vi "PromptWrite.vi"(8 "error in":errorcluster, 9 "time":timestamp, 10 "string":string, 11 "TerminalIn":T1) -> (0 "error out":errorcluster, 3 "TerminalOut":T1)   [LabVIEW 2021, in "LibDan.lvlib"]
uses:
  LibDan.lvlib
  TerminalDef.ctl
  <vilib>/Utility/config.llb/Config Data RefNum.ctl
  <vilib>/Utility/config.llb/NI_LVConfig.lvlib
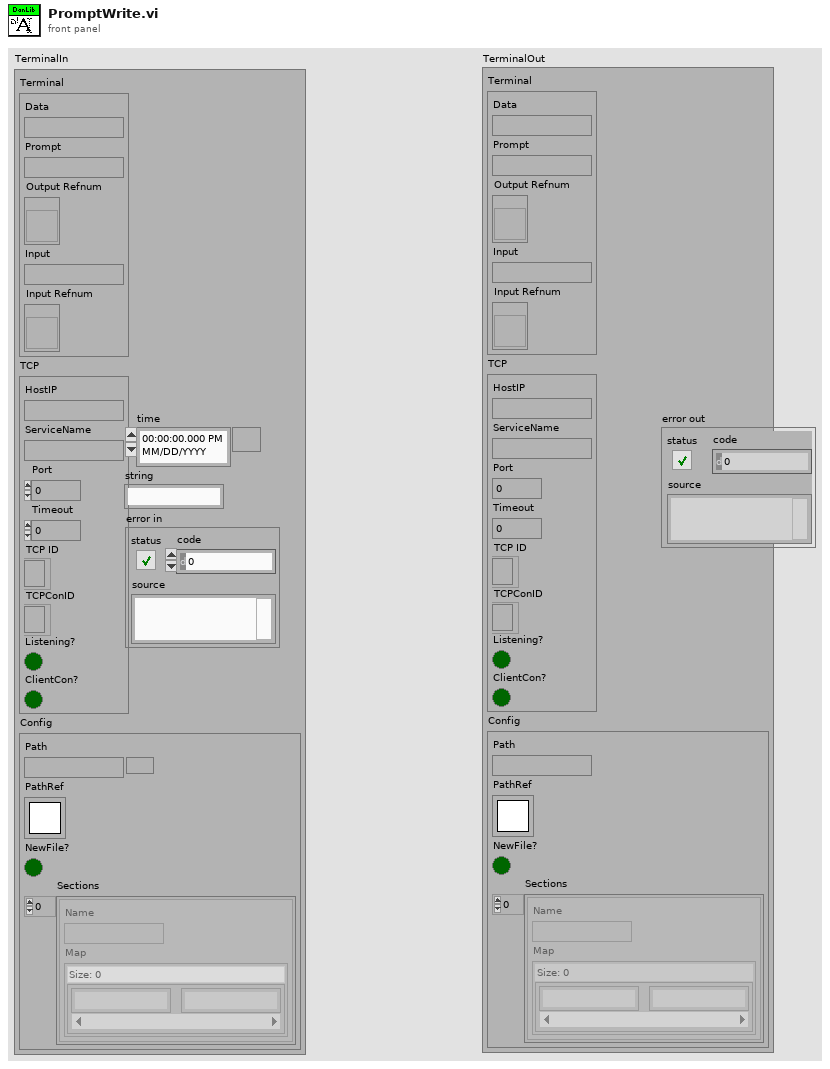
[diagram p1: front panel]
types:
  T1 = typedef "LibDan.lvlib/TerminalDef.ctl" = cluster{"Terminal":cluster{"Data":string, "Prompt":string, "Output Refnum":refnum<vi>, "Input":string, "Input Refnum":refnum<vi>}, "TCP":cluster{"HostIP":string, "ServiceName":string, "Port":u16, "Timeout":i32, "TCP ID":refnum<k5>, "TCPConID":refnum<k5>, "Listening?":bool, "ClientCon?":bool}, "Config":cluster{"Path":path, "PathRef":T2, "NewFile?":bool, "Sections":cluster{"Name":string, "Map":map{string, string}}[]}}
  T2 = typedef "NI_LVConfig.lvlib/Config Data RefNum.ctl" = refnum<k1>
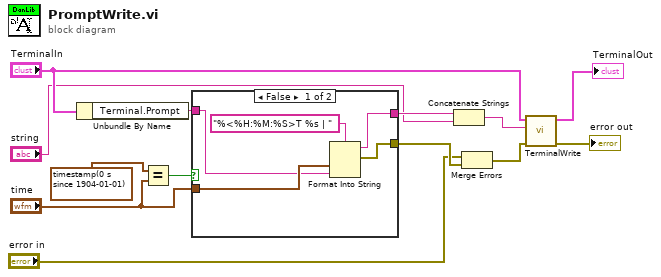
[diagram p0: block diagram]
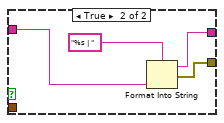
[diagram p2: hidden frame]
diagram:
  n1 = Unbundle By Name("TerminalIn") -> ("Terminal.Prompt"=w7:string)
  n2 = Equal?(x=timestamp(0 s since 1904-01-01), y="time") -> (x = y?=w11:bool)
  n3 = case shown="False" w11 {
    tunnel: [w18 w22] -> w2
    tunnel: "time" -> [w16 _]
    tunnel: w7 -> [w15 w20]
    tunnel: [w14 w19] -> w5
    frame False {
      n4 = Format Into String(format string="%<%H:%M:%S>T %s | ", w16, w15) -> (resulting string=w14:string, error out=w18:errorcluster)  [unwired: 2 in]
    }
    frame True {
      n5 = Format Into String(format string="%s | ", w20) -> (resulting string=w19:string, error out=w22:errorcluster)  [unwired: 2 in]
    }
  }
  n6 = Concatenate Strings(w5, "string") -> (w6:string)
  n7 = Merge Errors("error in", w2) -> (w3:errorcluster)
  n8 = call "TerminalWrite.vi"("error in"=w3, "string"=w6, "TerminalIn"="TerminalIn") -> ("error out"=→"error out":errorcluster, "TerminalOut"=→"TerminalOut":T1)  [unwired: 7 in]
